vi "RPC_DAQV3.vi"(7 "address":string[](array[string])=["192.168.10.20", "192.168.10.35"], 8 "error in (no error)":errorcluster, 9 "stop":bool=TRUE, 10 "save data":bool=TRUE, 11 "SMA mode":bool) -> (0 "error out 3":errorcluster, 2 "csv path":path=path "G:/tdc/2017/data/test_20250827_105458.csv", 3 "rate":dbl)   [LabVIEW 2017]
uses:
  gloabal.vi
  <vilib>/Utility/file.llb/Write Delimited Spreadsheet (DBL).vi
  <vilib>/Utility/file.llb/Write Delimited Spreadsheet (I64).vi
panel:
  out "Module NO":i32
  out "数组":errorcluster[](array[cluster])
  out "大小 5":i32=2
  out "大小 4":i32=2
  in  "cpu":i32=7
  out "大小 3":i32=2
  out "大小 2":i32=2
  out "大小":i32=2
  out "name (unnamed) 6":string="03E8"
  out "fine time":u64=3
  out "PAD NO":u64
  out "hitmap":u64 format="%08b"
  out "Array":string[](array[string])
  out "rpc trigger rate":u32[](array[numeric])=[0, 1000, 1000, 1000, 0, 0, 0, 0, 0, 0, 0, 1000, 1000, 0, 0, 0, 0, 0, 0, 0]
  out "event":u32[](array[numeric])=[0, 760, 1760, 1000, 0, 0, 0, 0, 0, 0, 0, 160, 160, 0, 0, 0, 0, 0, 0, 0]
  in  "calib_file":path=path "G:/tdc/2017/data/112_20250410_codeDensity.csv" caption="文件路径 （空时为对话框）"
  in  "use_calib_file":bool
  in  "coarse counter width":u16(ring) items=["29", "48"]
  out "error out 5":errorcluster
  in  "timeout":dbl=30000.0
  out "Out":u8=3 format="%.0x"
  in  "factor":i32=128
  in  "displayCR":bool=TRUE
  in  "Counter Setting":dbl=100000.0 format="%#_13g"
  in  "replace dat":bool
  in  "append csv":bool=TRUE
  out "element":string
  out "time":u64=1011186851 format="%x"
  in  "UDP Config":bool
  in  "data  path":path=path "G:/tdc/2017/data"
  out "cal 2":u64[](graph)=[12185147, 13185148, 14185150, 15185152, 16185153, 17185155, 18185157, 19185159, 20185160, 21185162, 22185164, 23185165, 24185167, 25185169, 26185170, 27185172, 28185174, 29185176, 30185177, 31185179, 32185181, 33185183, 34185184, 35185186, 36185188, 37185189, 38185191, 39185192, 40185194, 41185196, 42185198, 43185199, 44185201, 45185203, 46185205, 47185206, 48185208, 49185210, 50185212, 51185213, 52185215, 53185216, 54185218, 55185220, 56185222, 57185223, 58185225, 59185227, 60185229, 61185230, 62185232, 63185234, 64185235, 65185237, 66185239, 67185240, 68185242, 69185244, 70185246, 71185247, 72185249, 73185251, 74185253, 75185254, 76185256, 77185257, 78185259, 79185261, 80185263, 81185264, 82185266, 83185268, 84185270, 85185271, 86185273, 87185275, 88185276, 89185278, 90185280, 91185281, 92185283, 93185285, 94185287, 95185288, 96185290, 97185292, 98185294, 99185295, 100185297, 101185299, 102185300, 103185302, 104185304, 105185305, 106185307, 107185309, 108185311, 109185312, 110185314, 111185316, 112185317, 113185319, 114185321, 115185323, 116185324, 117185326, 118185328, 119185329, 120185331, 121185333, 122185335, 123185336, 124185338, 125185340, 126185341, 127185343, 128185344, 129185347, 130185348, 131185350, 132185351, 133185353, 134185355, 135185357, 136185358, 137185360, 138185362, 139185364, 140185365, 141185367, 142185368, 143185370, 144185372, 145185374, 146185375, 147185377, 148185379, 149185381, 150185382, 151185384, 152185386, 153185388, 154185389, 155185391, 156185392, 157185394, 158185396, 159185398, 160185399, 161185401, 162185403, 163185404, 164185406, 165185408, 166185410, 167185412, 168185413, 169185415, 170185416, 171185418, 172185420, 173185422, 174185423, 175185425, 176185427, 177185428, 178185430, 179185432, 180185433, 181185435, 182185437, 183185439, 184185440, 185185442, 186185444, 187185446, 188185447, 189185449, 190185451, 191185452, 192185454, 193185456, 194185457, 195185459, 196185461, 197185463, 198185464, 199185466, 200185468, 201185469, 202185471, 203185473, 204185475, 205185476, 206185478, 207185480, 208185481, 209185483, 210185485, 211185486, 212185488, 213185490, 214185492, 215185493, 216185495, 217185496, 218185498, 219185500, 220185502, 221185503, 222185505, 223185507, 224185509, 225185510, 226185512, 227185514, 228185516, 229185517, 230185519, 231185520, 232185522, 233185524, 234185526, 235185527, 236185529, 237185531, 238185533, 239185534, 240185536, 241185537, 242185539, 243185541, 244185543, 245185544, 246185546, 247185548, 248185550, 249185551, 250185553, 251185555, 252185556, 253185558, 254185560, 255185561, 256185563, 257185565, 258185567, 259185568, 260185570, 261185572, 262185573, 263185575, 264185577, 265185579, 266185580, 267185582, 268185584, 269185585, 270185587, 271185589, 272185591, 273185592, 274185594, 275185596, 276185597, 277185599, 278185601, 279185602, 280185604, 281185606, 282185608, 283185609, 284185611, 285185613, 286185615, 287185616, 288185618, 289185620, 290185621, 291185623, 372185761, 373185763, 374185765, 375185766, 376185768, 377185770, 378185772, 379185773, 380185775, 381185776, 382185778, 383185780, 384185782, 385185783, 386185785, 387185787, 388185788, 389185790, 390185792, 391185793, 392185795, 393185797, 394185799, 395185800, 396185802, 397185804, 398185806, 399185807, 400185809, 401185811, 402185812, 403185814, 404185816, 405185817, 406185819, 407185821, 408185823, 409185824, 410185826, 411185828, 412185829, 413185831, 414185833, 415185835, 416185836, 417185838, 418185840, 419185841, 420185843, 421185845, 422185847, 423185848, 424185850, 425185852, 426185853, 427185855, 428185857, 429185859, 430185860, 431185862, 432185864, 433185865, 434185867, 435185869, 436185871, 437185872, 438185874, 439185876, 440185877, 441185879, 442185881, 443185882, 444185884, 445185886, 446185887, 447185889, 448185891, 449185893, 450185894, 451185896, 452185898, 453185900, 454185901, 455185903, 456185904, 457185906, 458185908, 459185910, 460185911, 461185913, 462185915, 463185917, 464185918, 465185920, 466185921, 467185923, 468185925, 469185927, 470185928, 471185930, 472185932, 473185934, 474185935, 475185937, 476185939, 477185940, 478185942, 479185944, 480185946, 481185947, 482185949, 483185951, 484185952, 485185954, 486185956, 487185958, 488185959, 489185961, 490185963, 491185964, 492185966, 493185968, 494185969, 495185971, 496185973, 497185975, 498185976, 499185978, 500185980, 501185981, 502185983, 503185985, 504185987, 505185988, 506185990, 507185992, 508185993, 509185995, 510185997, 511185999, 512186000, 513186002, 514186004, 515186005, 516186007, 517186009, 518186011, 519186012, 520186014, 521186016, 522186017, 523186019, 524186021, 525186022, 526186024, 527186026, 528186028, 529186029, 530186031, 531186033, 532186034, 533186036, 534186038, 535186040, 536186041, 537186043, 538186045, 539186046, 540186048, 541186050, 542186052, 543186053, 544186055, 545186056, 546186058, 547186060, 548186062, 549186063, 550186065, 551186067, 552186069, 553186070, 554186072, 555186074, 556186076, 557186077, 558186079, 559186080, 560186082, 561186084, 562186086, 563186087, 564186089, 565186091, 566186093, 567186094, 568186096, 569186097, 570186099, 571186101, 572186103, 573186104, 574186106, 575186108, 576186110, 577186111, 578186113, 579186115, 580186116, 581186118, 582186120, 583186121, 584186123, 585186125, 586186127, 587186128, 588186130, 589186132, 590186133, 591186135, 592186137, 593186139, 594186140, 595186142, 596186144, 597186145, 598186147, 599186149, 600186151, 601186152, 602186154, 603186156, 604186157, 605186159, 606186160, 607186163, 608186164, 609186166, 610186167, 611186169, 692186308, 693186309, 694186311, 695186313, 696186315, 697186316, 698186318, 699186319, 700186321, 701186323, 702186325, 703186326, 704186328, 705186330, 706186332, 707186333, 708186335, 709186336, 710186338, 711186340, 712186342, 713186343, 714186345, 715186347, 716186349, 717186350, 718186352, 719186354, 720186356, 721186357, 722186359, 723186360, 724186362, 725186364, 726186366, 727186367, 728186369, 729186371, 730186373, 731186374, 732186376, 733186378, 734186379, 735186381, 736186383, 737186384, 738186386, 739186388, 740186390, 741186391, 742186393, 743186395, 744186397, 745186398, 746186400, 747186401, 748186403, 749186405, 750186407, 751186408, 752186410, 753186412, 754186414, 755186415, 756186417, 757186419, 758186420, 759186422, 760186424, 761186425, 762186427, 763186429, 764186431, 765186432, 766186434, 767186436, 768186438, 769186439, 770186441, 771186443, 772186444, 773186446, 774186448, 775186449, 776186451, 777186453, 778186455, 779186456, 780186458, 781186460, 782186461, 783186463, 784186465, 785186467, 786186468, 787186470, 788186472, 789186473, 790186475, 791186477, 792186478, 793186480, 794186482, 795186484, 796186485, 797186487, 798186489, 799186491, 800186492, 801186494, 802186496, 803186497, 804186499, 805186501, 806186502, 807186504, 808186506, 809186508, 810186509, 811186511, 812186513, 813186514, 814186516, 815186518, 816186519, 817186521, 818186523, 819186525, 820186526, 821186528, 822186530, 823186532, 824186533, 825186535, 826186536, 827186538, 828186540, 829186542, 830186543, 831186545, 832186547, 833186548, 834186550, 835186552, 836186554, 837186556, 838186557, 839186559, 840186560, 841186562, 842186564, 843186566, 844186567, 845186569, 846186571, 847186572, 848186574, 849186576, 850186577, 851186579, 852186581, 853186583, 854186584, 855186586, 856186588, 857186590, 858186591, 859186593, 860186595, 861186596, 862186598, 863186600, 864186601, 865186603, 866186605, 867186607, 868186608, 869186610, 870186612, 871186613, 872186615, 873186617, 874186619, 875186620, 876186622, 877186624, 878186625, 879186627, 880186629, 881186631, 882186632, 883186634, 884186636, 885186637, 886186639, 887186641, 888186643, 889186644, 890186646, 891186648, 892186649, 893186651, 894186653, 895186655, 896186656, 897186658, 898186660, 899186661, 900186663, 901186664, 902186666, 903186668, 904186670, 905186672, 906186673, 907186675, 908186677, 909186678, 910186680, 911186682, 912186684, 913186685, 914186687, 915186688, 916186690, 917186692, 918186694, 919186695, 920186697, 921186699, 922186701, 923186702, 924186704, 925186706, 926186707, 927186709, 928186711, 929186712, 930186714, 931186716]
  in  "Thresholds (mV)":dbl[](array[numeric])=[580.0, 580.0, 580.0, 580.0, 600.0, 600.0, 600.0, 600.0, 580.0, 580.0, 600.0, 600.0, 600.0, 600.0, 600.0, 600.0, 580.0, 580.0, 600.0, 600.0, 600.0, 600.0, 600.0, 600.0, 580.0, 580.0, 600.0, 600.0, 600.0, 600.0, 600.0, 600.0, 600.0, 600.0, 600.0, 600.0, 600.0, 600.0, 600.0, 600.0, 600.0, 600.0, 600.0, 600.0, 600.0, 600.0, 600.0, 600.0, 600.0, 600.0, 600.0, 600.0, 600.0, 600.0, 600.0, 600.0, 600.0, 600.0, 600.0, 600.0, 600.0, 600.0, 600.0, 600.0]
  out "error out 2":errorcluster
  in  "display":bool=TRUE
  in  "Thresholds":dbl=-0.03
  in  "one key for threshold":bool=TRUE
  in  "RST":bool
  in  "通道数量":i32=10
  out "Cal Table":u32[](array[numeric])
  in  "channel for cal":i32
  out "Strip NO":u64
  out "Calibration Counter":i32=3364
  out "Event index":i32=97959
  out "cal":i64[](graph)
  out "error out":errorcluster
  out "appended path":path=path "G:/tdc/2017/data/test_20250827_105458.dat"
  in  "filename":string="test"
  in  "Events":i32=110000 min=1
  in  "timeout (ms)":i32=10000
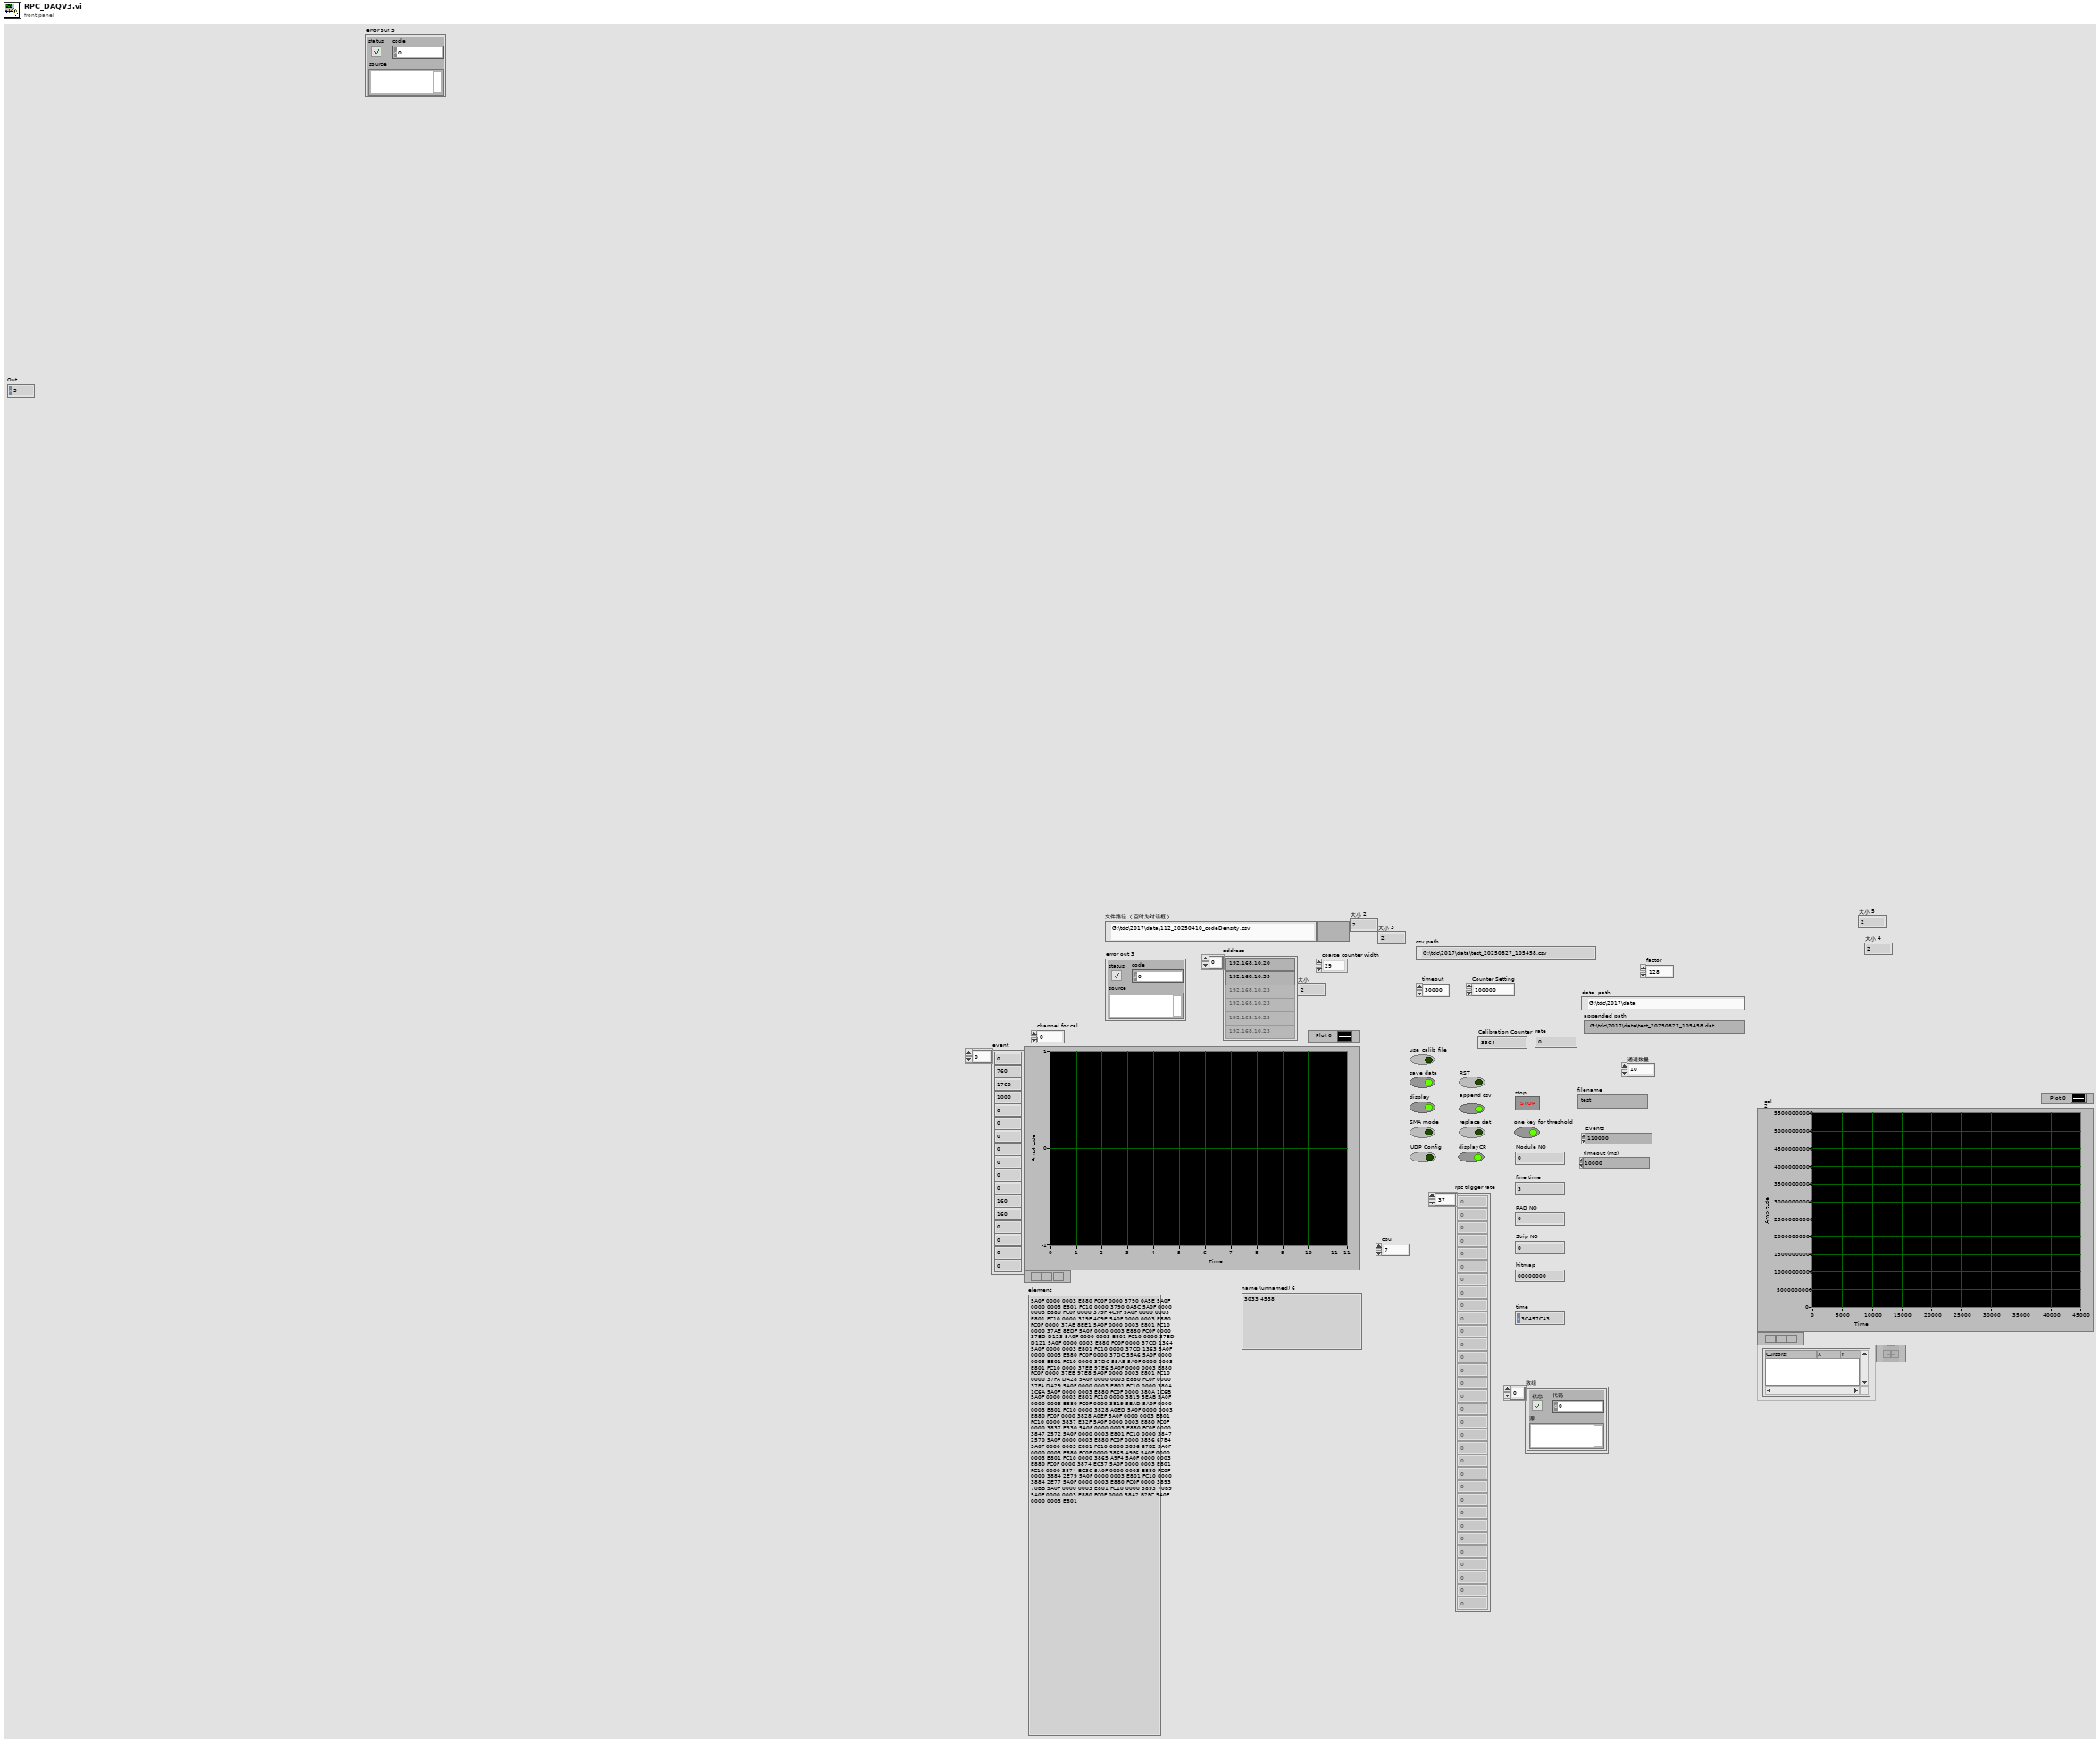
[diagram p1: front panel]
types:
  T1 = enum16{"open", "replace", "create", "open or create", "replace or create", "replace or create with confirmation"}
  T2 = enum16{"big-endian, network order", "native, host order", "little-endian"}
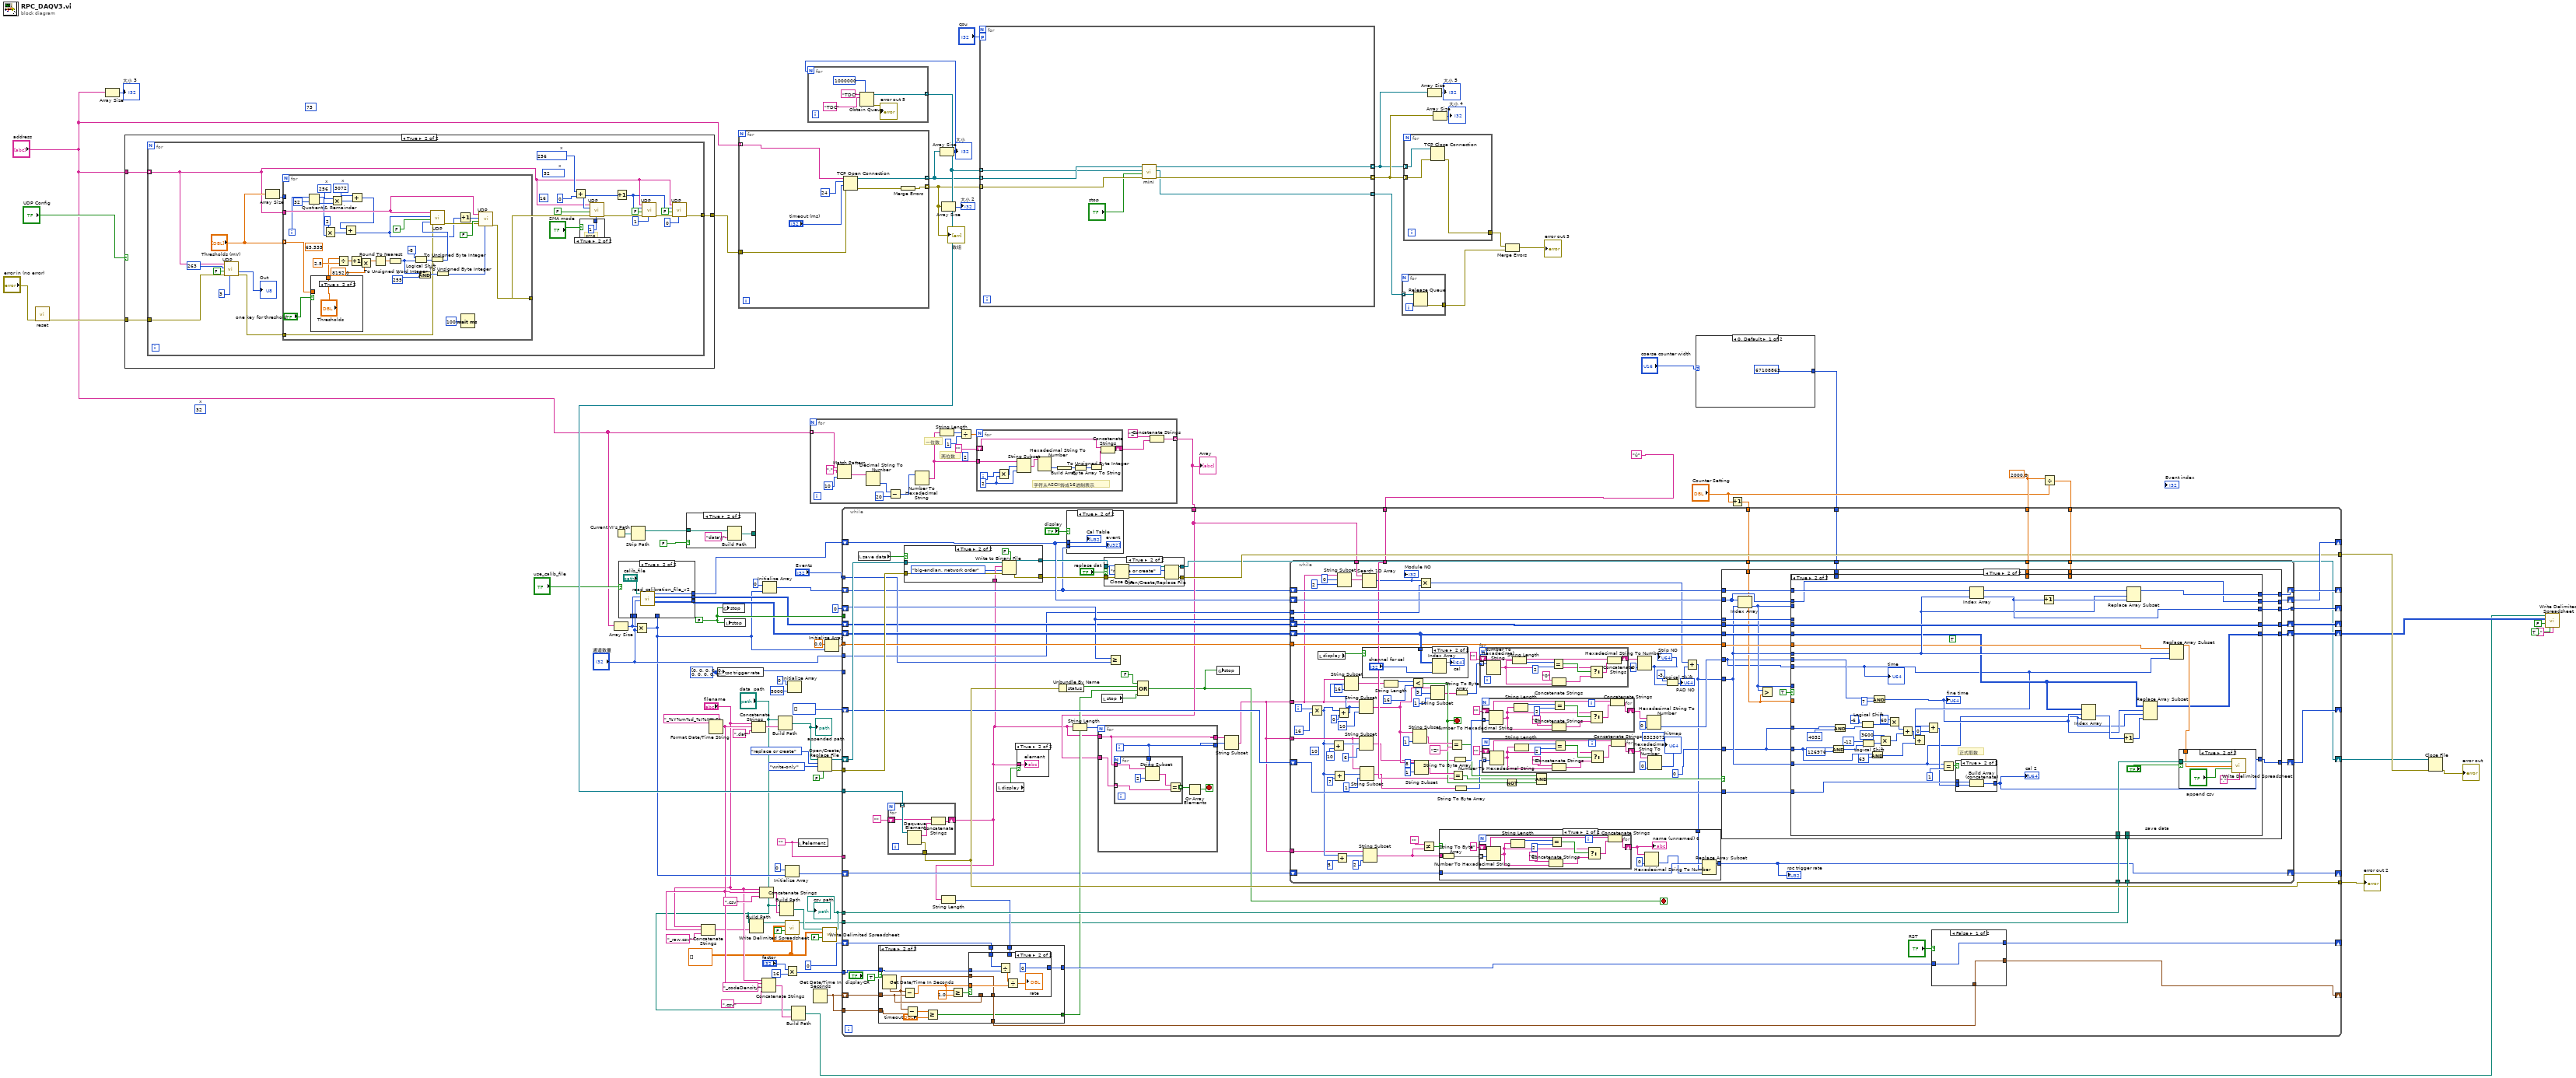
[diagram p0: block diagram]
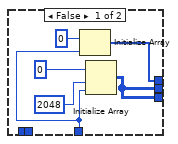
[diagram p2: hidden frame]
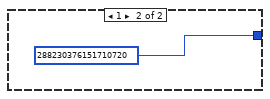
[diagram p3: hidden frame]
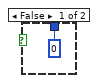
[diagram p5: hidden frame]
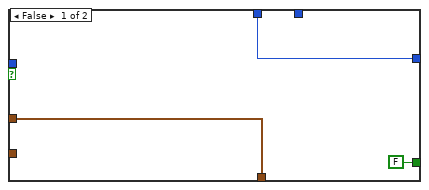
[diagram p11: hidden frame]
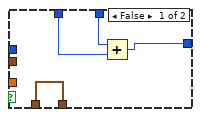
[diagram p12: hidden frame]
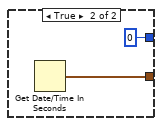
[diagram p14: hidden frame]
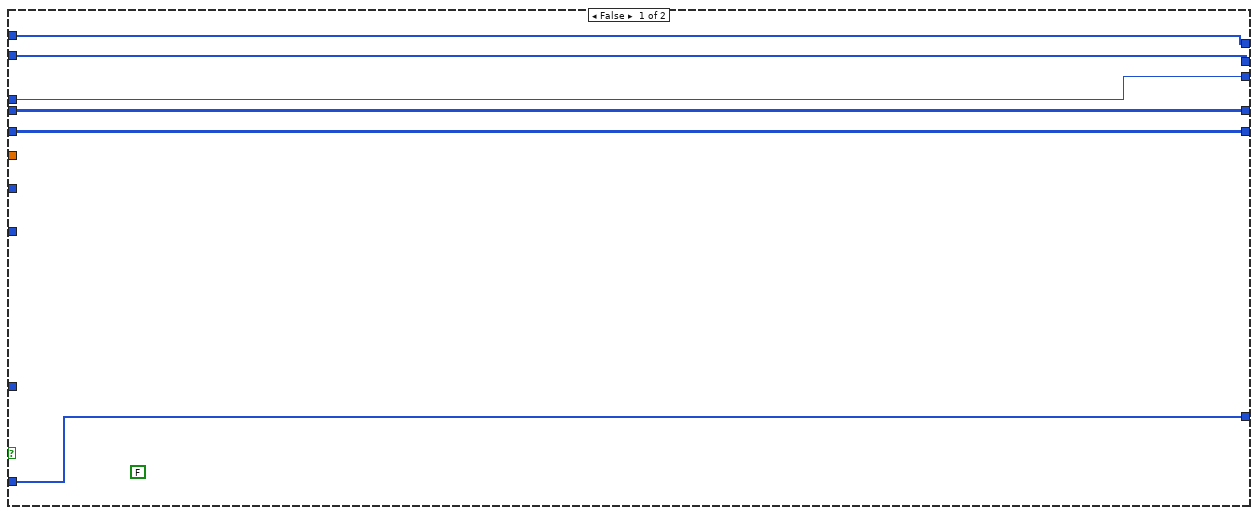
[diagram p17: hidden frame]
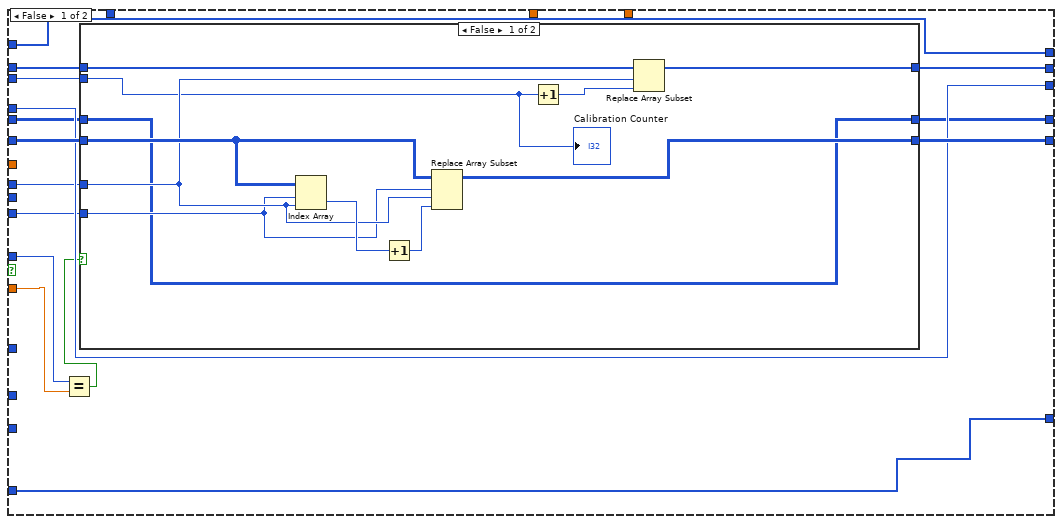
[diagram p18: hidden frame]
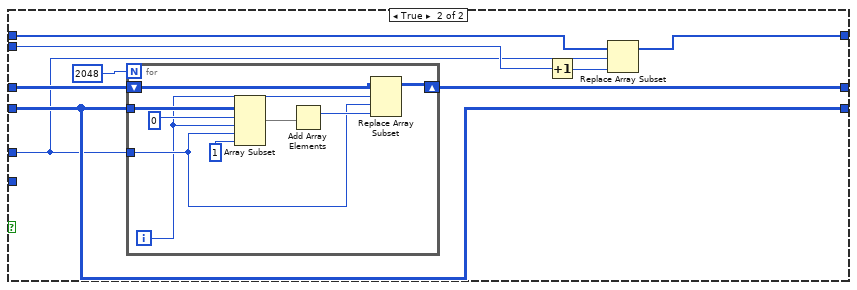
[diagram p19: hidden frame]
diagram:
  w24 = ""
  w25 = u32[] [0, 0, 0, 0, 0, 0, 0, 0, 0, 0, 0, 0, 0, 0, 0, 0, 0, 0, 0, 0, 0, 0, 0, 0, 0, 0, 0, 0, 0, 0, 0, 0, 0, 0, 0, 0, 0, 0, 0, 0, 0, 0, 0, 0, 0, 0, 0, 0, 0, 0, 0, 0, 0, 0, 0, 0, 0, 0, 0, 0, 0, 0, 0, 0] ("pmt trigger rate")
  (unwired) u32 73 ("Address")
  w56 = 2000.0 ("x")
  (unwired) u16 32  # x
  w38 = FALSE ("stop")
  w18 = dbl[][] [] ("2D data")
  n1 = call "reset.vi"("error in (no error)"="error in (no error)") -> ("error out"=w12:errorcluster)  [unwired: 10 in]
  n2 = Array Size(array="address") -> (size(s)=→"大小 3":i32)
  n3 = case shown="True" "UDP Config" {
    tunnel: "address" -> [_ w94]
    tunnel: [_ w95] -> w42
    tunnel: w12 -> [_ w93]
    frame False {
    }
    frame True {
      n4 = for {
        tunnel: [w101] -> w95
        tunnel: w94 -> [w99] mode=indexing
        tunnel: w93 -> [w96]
        (unwired) u16 32  # x
        (unwired) u32 16 ("Address")
        w112 = u16 256  # x
        n5 = call "UDP.vi"("In"=u8 3, "error in (no error)"=w96, "Read (TRUE)"=FALSE, "Address"=u32 263, "IP address"=w99) -> ("error out"=w107:errorcluster, "Out"=→"Out":u8)  [unwired: 3 in, 1 out]
        n6 = Array Size(array="Thresholds (mV)") -> (size(s)=w115:i32)
        n7 = for {
          tunnel: w99 -> [w151]
          tunnel: "Thresholds (mV)" -> [w138] mode=indexing
          tunnel: [w141] -> w118
          tunnel: w115 -> [_]
          tunnel: w107 -> [w125]
          i -> [w133]
          (unwired) 65.535 ("y")
          w134 = u16 3072  # x
          w135 = u16 256  # x
          w147 = u16 255  # x
          n8 = Quotient & Remainder(x=w133, y=32) -> (x-y*floor(x/y)=w127:i32, floor(x/y)=w136:i32)
          n9 = case shown="True" "one key for threshold" {
            tunnel: [w157 "Thresholds"] -> w139
            tunnel: w138 -> [w157 _]
            frame False {
            }
            frame True {
            }
          }
          n10 = Multiply(x=2, y=w127) -> (x*y=w128:i32)
          n11 = Multiply(x=w135, y=w136) -> (x*y=w130:i32)
          n12 = Divide(x=w139, y=2.5) -> (x/y=w154:dbl)
          n13 = Increment(x=w154) -> (x+1=w124:dbl)
          n14 = Add(x=w134, y=w130) -> (x+y=w129:i32)
          n15 = Add(x=w129, y=w128) -> (x+y=w132:i32)
          n16 = Multiply(x=w124, y=8192.0) -> (x*y=w123:dbl)
          n17 = Round To Nearest(number=w123) -> (nearest integer value=w152:dbl)
          n18 = To Unsigned Word Integer(number=w152) -> (unsigned 16bit integer=w143:u16)
          n19 = Logical Shift(y=i16 -8, x=w143) -> (x << y=w149:u16)
          n20 = And(x=w143, y=w147) -> (x .and. y?=w146:u16)
          n21 = To Unsigned Byte Integer(number=w149) -> (unsigned 8bit integer=w148:u8)
          n22 = call "UDP.vi"("In"=w148, "error in (no error)"=w125, "Read (TRUE)"=FALSE, "Address"=w132, "IP address"=w151) -> ("error out"=w142:errorcluster)  [unwired: 3 in, 2 out]
          n23 = To Unsigned Byte Integer(number=w146) -> (unsigned 8bit integer=w145:u8)
          n24 = Increment(x=w132) -> (x+1=w131:i32)
          n25 = Wait (ms)(milliseconds to wait=u32 100) -> ()  [unwired: 1 out]
          n26 = call "UDP.vi"("In"=w145, "error in (no error)"=w142, "Read (TRUE)"=FALSE, "Address"=w131, "IP address"=w151) -> ("error out"=w141:errorcluster)  [unwired: 3 in, 2 out]
        }
        n27 = Add(x=w112, y=u32 0 ("Address")) -> (x+y=w105:u32)
        n28 = case shown="True" "SMA mode" {
          tunnel: [u8 0 ("In") u8 1 ("In")] -> w117
          frame False {
          }
          frame True {
            # "sma"
          }
        }
        n29 = call "UDP.vi"("In"=w117, "error in (no error)"=w118, "Read (TRUE)"=FALSE, "Address"=w105, "IP address"=w99) -> ("error out"=w106:errorcluster)  [unwired: 3 in, 2 out]
        n30 = Increment(x=w105) -> (x+1=w98:u32)
        n31 = call "UDP.vi"("In"=u8 1, "error in (no error)"=w106, "Read (TRUE)"=FALSE, "Address"=w98, "IP address"=w99) -> ("error out"=w102:errorcluster)  [unwired: 3 in, 2 out]
        n32 = call "UDP.vi"("In"=u8 0, "error in (no error)"=w102, "Read (TRUE)"=FALSE, "Address"=w98, "IP address"=w99) -> ("error out"=w101:errorcluster)  [unwired: 3 in, 2 out]
      }
    }
  }
  n33 = Current VI's Path() -> (path=w87:path)
  n34 = Array Size(array="address") -> (size(s)=w30:i32)
  n35 = Strip Path(path=w87) -> (stripped path=w86:path)  [unwired: 1 out]
  n36 = Multiply(x=w30, y="通道数量") -> (x*y=w27:i32)
  n37 = case shown="True" "use_calib_file" {
    tunnel: w27 -> [w162 _]
    tunnel: [w159 w170] -> w33
    tunnel: [w159 w169] -> w32
    tunnel: [w160 w168] -> w31
    tunnel: w30 -> [_ w167]
    tunnel: "通道数量" -> [_ w166]
    frame False {
      n38 = Initialize Array(u32 0 ("element"), w162) -> (w160:u32[])
      n39 = Initialize Array(u32 0 ("element"), 2048 ("dimension size"), w162) -> (w159:u32[][])
    }
    frame True {
      n40 = call "read_calibration_file_v2.vi"("通道数量"=w166, "板子数量"=w167, "file path (dialog if empty)"="calib_file") -> ("code_density"=w170:i64[][], "accumulation"=w169:u32[][], "Cal Table"=w168:u32[])  [unwired: 5 in, 1 out]
    }
  }
  n41 = case shown="True" FALSE {
    tunnel: w86 -> [w171 w173]
    tunnel: [w171 w172] -> _
    frame False {
    }
    frame True {
      n42 = Build Path(base path=w173, name or relative path="data\\") -> (appended path=w172:path)
    }
  }
  n43 = Format Date/Time String(time format string (%c)="_%Y%m%d_%I%M%S") -> (date/time string=w22:string)  [unwired: 2 in]
  n44 = Concatenate Strings("filename", w22, "_raw.csv") -> (w20:string)
  n45 = local write "rpc trigger rate"(w25) -> ()
  n46 = global write "gloabal.vi" "stop"(w38) -> ()
  n47 = local write "stop"(w38) -> ()
  n48 = for {
    tunnel: "address" -> [w180] mode=indexing
    tunnel: [w179] -> w10 mode=indexing
    tunnel: [w177] -> w11 mode=indexing
    tunnel: w42 -> [w176]
    n49 = TCP Open Connection(address=w180, remote port or service name=u16 24 ("port"), timeout ms (60000)="timeout (ms)", error in (no error)=w176) -> (connection ID=w179:refnum<k5>, error out=w178:errorcluster)  [unwired: 1 in]
    n50 = Merge Errors(w178) -> (w177:errorcluster)
  }
  "数组" <- w11
  n51 = Build Path(base path="data  path", name or relative path=w20) -> (appended path=w15:path)
  n52 = Concatenate Strings("filename", w22, ".dat") -> (w85:string)
  n53 = Concatenate Strings("filename", w22, ".csv") -> (w75:string)
  n54 = Concatenate Strings("filename", w22, "_codeDensity" ("string"), ".csv") -> (w68:string)
  n55 = Initialize Array(u32 0 ("element"), w27) -> (w74:u32[])
  n56 = Build Path(base path="data  path", name or relative path=w85) -> (appended path=w84:path)
  "appended path" <- w84
  n57 = Build Path(base path="data  path", name or relative path=w75) -> (appended path=w73:path)
  n58 = Initialize Array(u32 0 ("element"), w27) -> (w26:u32[])
  n59 = call-poly <vilib>:"Write Delimited Spreadsheet.vi"("file path (dialog if empty)"=w15, "2D data"=w18, "append to file? (new file:F)"=FALSE) -> ("new file path (Not A Path if cancelled)"=w16:path)  [unwired: 11 in, 1 out]
  n60 = Multiply(x="factor", y=16) -> (x*y=w49:i32)
  n61 = Initialize Array(u32 0 ("element"), 5000 ("dimension size")) -> ()  [unwired: 1 out]
  n62 = Build Path(base path="data  path", name or relative path=w68) -> (appended path=w65:path)
  n63 = local write "element"(w24) -> ()
  n64 = for {
    tunnel: [w183] -> w46 mode=indexing
    tunnel: "address" -> [w182] mode=indexing
    (unwired) 2 ("y")
    # "一位数"
    # "两位数"
    n65 = Match Pattern(string=w182, regular expression="." ("search string"), offset (0)=10) -> (after substring=w189:string)  [unwired: 3 out]
    n66 = Decimal String To Number(string=w189) -> (number=w186:i32)  [unwired: 2 in, 1 out]
    n67 = Subtract(x=w186, y=20) -> (x-y=w185:i32)
    n68 = Number To Hexadecimal String(2:w185) -> (0:w188:string)  [unwired: 1 in]
    n69 = String Length(string=w188) -> (length=w194:i32)
    n70 = Divide(x=w194, y=1) -> (x/y=w195:dbl)
    n71 = for {
      N: w195 -> [_]
      shift-right: [w207] -> w184
      shift-left: "" ("format string") -> [w206]
      tunnel: w188 -> [w197]
      i -> [w205]
      w199 = 2 ("y")
      # "字符从ASCII转成16进制表示"
      n72 = Multiply(x=w205, y=w199) -> (x*y=w198:i32)
      n73 = String Subset(string=w197, offset (0)=w198, length (rest)=w199) -> (substring=w200:string)
      n74 = Hexadecimal String To Number(string=w200) -> (number=w204:u32)  [unwired: 2 in, 1 out]
      n75 = Build Array(w204) -> (w203:u32[])
      n76 = To Unsigned Byte Integer(number=w203) -> (unsigned 8bit integer=w202:u8[])
      n77 = Byte Array To String(unsigned byte array=w202) -> (string=w201:string)
      n78 = Concatenate Strings(w206, w201) -> (w207:string)
    }
    n79 = Concatenate Strings("Z", w184) -> (w183:string)
  }
  "Array" <- w46
  n80 = Get Date/Time In Seconds() -> (seconds since 1Jan1904=w45:timestamp)
  n81 = Open/Create/Replace File(file path (use dialog)=w84, operation (0:open)=T1."replace or create", access (0:read/write)=enum16{"read/write", "read-only", "write-only"}."write-only", disable buffering (F)=FALSE) -> (refnum out=w89:refnum<file>, error out=w88:errorcluster)  [unwired: 2 in, 1 out]
  n82 = call-poly <vilib>:"Write Delimited Spreadsheet.vi"("file path (dialog if empty)"=w73, "2D data"=w18, "append to file? (new file:F)"=FALSE) -> ("new file path (Not A Path if cancelled)"=w37:path)  [unwired: 11 in, 1 out]
  "csv path" <- w37
  n83 = Initialize Array(0.0, w27) -> (w61:dbl[])
  n84 = Array Size(array=w10) -> (size(s)=w2:i32)
  "大小" <- w2
  n85 = for {
    N: w2 -> [_]
    tunnel: [w208] -> w43 mode=indexing
    n86 = Obtain Queue(max queue size (-1, unlimited)=1000000, name (unnamed)="TDC", element data type="TDC" ("name (unnamed)")) -> (queue out=w208:refnum<queue>, error out=→"error out 5":errorcluster)  [unwired: 2 in, 1 out]
  }
  n87 = Array Size(array=w11) -> (size(s)=→"大小 2":i32)
  n88 = for {
    tunnel: w10 -> [w219] mode=indexing
    tunnel: w11 -> [w218] mode=indexing
    tunnel: [w217] -> w3 mode=indexing
    tunnel: [w216] -> w5 mode=indexing
    tunnel: w43 -> [w215] mode=indexing
    tunnel: [w214] -> w44 mode=indexing
    workers-P: "cpu" -> [_]
    n89 = call "mini.vi"("error in (no error)"=w218, "stop"="stop", "queue out 2"=w215, "connection ID 2"=w219) -> ("error out 3"=w216:errorcluster, "queue out"=w214:refnum<queue>, "connection ID"=w217:refnum<k5>)  [unwired: 5 in]
  }
  n90 = for {
    tunnel: w44 -> [w221] mode=indexing
    tunnel: [w220] -> w40
    n91 = Release Queue(queue=w221) -> (error out=w220:errorcluster)  [unwired: 2 in, 2 out]
  }
  n92 = for {
    tunnel: w3 -> [w224] mode=indexing
    tunnel: w5 -> [w223] mode=indexing
    tunnel: [w222] -> w41
    n93 = TCP Close Connection(connection ID=w224, error in (no error)=w223) -> (error out=w222:errorcluster)  [unwired: 1 in, 1 out]
  }
  n94 = Array Size(array=w3) -> (size(s)=→"大小 5":i32)
  n95 = Array Size(array=w5) -> (size(s)=→"大小 4":i32)
  n96 = Merge Errors(w41, w40) -> (→"error out 3":errorcluster)
  n97 = case shown="0, Default" "coarse counter width" {
    tunnel: [u64 67108863 ("port") u64 288230376151710720 ("port")] -> w35
    frame 0, Default {
    }
    frame 1 {
    }
  }
  n98 = Increment(x="Counter Setting") -> (x+1=w52:dbl)
  n99 = Divide(x=w56, y="Counter Setting") -> (x/y=w55:dbl)
  n100 = while {
    tunnel: w88 -> [w285]
    tunnel: [w266] -> w62
    tunnel: [w255] -> w81
    shift-right: [w282] -> w66
    shift-left: w33 -> [w283]
    tunnel: "Events" -> [w280]
    shift-right: [w279] -> _
    shift-left: w74 -> [w233]
    shift-right: [w278] -> _
    shift-left: u32 0 ("element") -> [w277]
    shift-right: [w276] -> _
    shift-left: w31 -> [w268]
    shift-right: [w270] -> _
    shift-left: w32 -> [w275]
    tunnel: w37 -> [w262]
    shift-right: [w274] -> _
    shift-left: 0 -> [w249]
    shift-right: [w272] -> _
    shift-left: w45 -> [w271]
    tunnel: w38 -> [_]
    tunnel: w43 -> [w267]
    shift-right: [w263] -> _
    shift-left: u64[] [] -> [w264]
    tunnel: w46 -> [w237]
    tunnel: w56 -> [w260]
    tunnel: w55 -> [w259]
    shift-right: [w254] -> w54
    shift-left: w89 -> [w284]
    tunnel: w52 -> [w253]
    tunnel: w49 -> [w246]
    tunnel: "ü" ("format string") -> [w244]
    tunnel: w45 -> [w243]
    tunnel: "通道数量" -> [w238]
    tunnel: w35 -> [w234]
    shift-right: [w230] -> _
    shift-left: w26 -> [w231]
    tunnel: w25 -> [_]
    tunnel: w24 -> [_]
    tunnel: w16 -> [w229]
    tunnel: w61 -> [w281]
    stop <- w236 stop-if-true
    n101 = local read "save data"() -> (w248:bool)
    n102 = for {
      tunnel: w267 -> [w290] mode=indexing
      tunnel: [w289] -> w266
      shift-right: [w288] -> w227
      shift-left: "" -> [w286]
      n103 = Dequeue Element(queue=w290) -> (element=w287:string, error out=w289:errorcluster)  [unwired: 2 in, 2 out]
      n104 = Concatenate Strings(w286, w287) -> (w288:string)
    }
    n105 = case shown="True" w248 {
      tunnel: w285 -> [w303 w311]
      tunnel: w284 -> [w304 w310]
      tunnel: w227 -> [_ w308]
      tunnel: [w304 w307] -> w258
      tunnel: [w303 w306] -> w256
      frame False {
      }
      frame True {
        n106 = Write to Binary File(file (use dialog)=w310, data=w308, error in=w311, 5:FALSE ("prepend array or string size? (T)"), 9:T2."big-endian, network order" ("byte order (0:big-endian, network order)")) -> (refnum out=w307:refnum<file>, error out=w306:errorcluster)  [unwired: 1 in, 1 out]
      }
    }
    n107 = String Length(string=w227) -> (length=w250:i32)
    n108 = case shown="True" TRUE {
      tunnel: w271 -> [w323 w333]
      tunnel: [w323 w334] -> w252
      tunnel: w249 -> [w322 w332]
      tunnel: w250 -> [_ w331]
      tunnel: [w322 w330] -> w251
      tunnel: w246 -> [_ w329]
      tunnel: w243 -> [_ w327]
      tunnel: [FALSE w324] -> w242
      frame False {
      }
      frame True {
        n109 = Get Date/Time In Seconds() -> (seconds since 1Jan1904=w328:timestamp)
        n110 = Subtract(x=w328, y=w333) -> (x-y=w336:dbl)
        n111 = Subtract(x=w328, y=w327) -> (x-y=w326:dbl)
        n112 = Greater Or Equal?(x=w326, y="timeout") -> (x >= y?=w324:bool)
        n113 = Greater Or Equal?(x=w336, y=1.0) -> (x >= y?=w337:bool)
        n114 = case shown="True" w337 {
          tunnel: w336 -> [_ w348]
          tunnel: w328 -> [_ w346]
          tunnel: [w341 w346] -> w334
          tunnel: w333 -> [w341 _]
          tunnel: w332 -> [w340 w343]
          tunnel: w331 -> [w339 _]
          tunnel: [w338 0] -> w330
          tunnel: w329 -> [_ w342]
          frame False {
            n115 = Add(x=w339, y=w340) -> (x+y=w338:i32)
          }
          frame True {
            n116 = Divide(x=w343, y=w342) -> (x/y=w345:dbl)
            n117 = Divide(x=w345, y=w348) -> (x/y=→"rate":dbl)
          }
        }
      }
    }
    n118 = local read "display"() -> (w247:bool)
    n119 = case shown="True" w247 {
      tunnel: w227 -> [_ w302]
      frame False {
      }
      frame True {
        "element" <- w302
      }
    }
    n120 = Unbundle By Name(w266) -> ("status"=w265:bool)
    n121 = case shown="True" "display" {
      tunnel: w268 -> [_ w350]
      tunnel: w233 -> [_ w349]
      frame False {
      }
      frame True {
        "Cal Table" <- w350
        "event" <- w349
      }
    }
    n122 = String Length(string=w227) -> (length=w241:i32)
    n123 = for {
      N: w241 -> [_]
      tunnel: w227 -> [w295]
      tunnel: [w295] -> w240
      tunnel: [w294] -> w239
      tunnel: w237 -> [w293]
      i -> [w294]
      stop <- w292 stop-if-true
      n124 = for {
        tunnel: [w300] -> w291 mode=indexing
        tunnel: w295 -> [w299]
        tunnel: w294 -> [w298]
        tunnel: w293 -> [w296] mode=indexing
        n125 = String Subset(string=w299, offset (0)=w298, length (rest)=2 ("length (rest)")) -> (substring=w297:string)
        n126 = Equal?(x=w297, y=w296) -> (x = y?=w300:bool)
      }
      n127 = Or Array Elements(Boolean array=w291) -> (logical OR=w292:bool)
    }
    n128 = local read "stop"() -> (w235:bool)
    n129 = case shown="True" "replace dat" {
      tunnel: w258 -> [w313 w319]
      tunnel: [w313 w318] -> w254
      tunnel: w256 -> [w312 w315]
      tunnel: [w312 w314] -> w255
      frame False {
      }
      frame True {
        n130 = Close File(refnum=w319, error in=w315) -> (path=w320:path, error out=w316:errorcluster)
        n131 = Open/Create/Replace File(file path (use dialog)=w320, error in=w316, operation (0:open)=T1."replace or create") -> (refnum out=w318:refnum<file>, error out=w314:errorcluster)  [unwired: 3 in, 1 out]
      }
    }
    n132 = Greater Or Equal?(x=w277, y=w280) -> ()  [unwired: 1 out]
    n133 = Compound Arithmetic op=OR(FALSE ("x"), w265, w242, w235) -> (w236:bool)
    n134 = global write "gloabal.vi" "stop"(w236) -> ()
    n135 = String Subset(string=w240, offset (0)=w239) -> (substring=w232:string)  [unwired: 1 in]
    n136 = while {
      tunnel: w232 -> [w366]
      shift-right: [w442] -> w282
      shift-left: w283 -> [w441]
      shift-right: [w437] -> w279
      shift-left: w233 -> [w436]
      tunnel: [w435] -> w278
      tunnel: w277 -> [w434]
      shift-right: [w432] -> w276
      shift-left: w268 -> [w433]
      tunnel: w262 -> [w430]
      shift-right: [w429] -> w270
      shift-left: w275 -> [w401]
      shift-right: [w426] -> w263
      shift-left: w264 -> [w427]
      tunnel: w232 -> [w395]
      tunnel: w260 -> [w407]
      tunnel: w259 -> [w406]
      tunnel: w253 -> [w400]
      tunnel: w244 -> [w390]
      tunnel: w238 -> [w381]
      tunnel: w237 -> [w380]
      tunnel: w234 -> [w378]
      tunnel: w232 -> [w371]
      shift-right: [w363] -> w230
      shift-left: w231 -> [w373]
      tunnel: w229 -> [w368]
      tunnel: w281 -> [w440]
      i -> [w443]
      stop <- w403 stop-if-true
      (unwired) 10 ("length (rest)")
      (unwired) u64 8323072 ("port")
      n137 = Multiply(x=w443, y=16 ("length (rest)")) -> (x*y=w374:i32)
      n138 = local read "display"() -> (w428:bool)
      n139 = Add(x=w374, y=10 ("length (rest)")) -> (x+y=w418:i32)
      n140 = Add(x=w374, y=7 ("length (rest)")) -> (x+y=w397:i32)
      n141 = Add(x=w374, y=5 ("length (rest)")) -> (x+y=w376:i32)
      n142 = Add(x=w374, y=0 ("length (rest)")) -> (x+y=w405:i32)
      n143 = String Subset(string=w366, offset (0)=0, length (rest)=2 ("length (rest)")) -> (substring=w355:string)
      n144 = String Subset(string=w366, offset (0)=w405, length (rest)=16 ("y")) -> (substring=w358:string)
      n145 = String Subset(string=w366, offset (0)=w405, length (rest)=10 ("length (rest)")) -> (substring=w365:string)
      n146 = String Subset(string=w395, offset (0)=w418, length (rest)=6 ("length (rest)")) -> (substring=w364:string)
      n147 = String Subset(string=w395, offset (0)=w397, length (rest)=1 ("length (rest)")) -> (substring=w386:string)
      n148 = Search 1D Array(1D array=w380, element=w355) -> (index of element=w382:i32)  [unwired: 1 in]
      "Module NO" <- w382
      n149 = case shown="True" w428 {
        tunnel: w441 -> [_ w488]
        frame False {
        }
        frame True {
          n150 = Index Array(array=w488, index (col)="channel for cal") -> (element=→"cal":i64[])  [unwired: 1 in]
        }
      }
      n151 = String Subset(string=w371, offset (0)=w376, length (rest)=2 ("length (rest)")) -> (substring=w356:string)
      n152 = String Length(string=w358) -> (length=w439:i32)
      n153 = Less?(x=w439, y=16) -> (x < y?=w403:bool)
      n154 = String Subset(string=w365, length (rest)=1 ("length (rest)")) -> (substring=w423:string)  [unwired: 1 in]
      n155 = String Subset(string=w365, offset (0)=8, length (rest)=1 ("length (rest)")) -> (substring=w408:string)
      n156 = Multiply(x=w382, y=w381) -> (x*y=w379:i32)
      n157 = Not Equal?(x="", y=w356) -> (x != y?=w370:bool)
      n158 = String Subset(string=w365, offset (0)=9, length (rest)=1 ("length (rest)")) -> (substring=w387:string)
      n159 = Equal?(x=w423, y="Z" ("format string")) -> (x = y?=w409:bool)
      n160 = Equal?(x=w408, y=w390) -> (x = y?=w362:bool)
      n161 = String To Byte Array(string=w364) -> (unsigned byte array=w415:u8[])
      n162 = String To Byte Array(string=w386) -> (unsigned byte array=w391:u8[])
      n163 = String To Byte Array(string=w387) -> (unsigned byte array=w444:u8[])
      n164 = for {
        shift-right: [w622] -> w412
        shift-left: "" ("format string") -> [w619]
        tunnel: w444 -> [w623] mode=indexing
        n165 = Number To Hexadecimal String(2:w623) -> (0:w615:string)  [unwired: 1 in]
        n166 = String Length(string=w615) -> (length=w621:i32)
        n167 = Equal?(x=w621, y=2) -> (x = y?=w618:bool)
        n168 = Concatenate Strings("0" ("format string"), w615) -> (w617:string)
        n169 = Select(t=w615, s=w618, f=w617) -> (s? t:f=w614:string)
        n170 = Concatenate Strings(w619, w614) -> (w622:string)
      }
      n171 = for {
        shift-right: [w484] -> w413
        shift-left: "" ("format string") -> [w476]
        tunnel: w415 -> [w485] mode=indexing
        n172 = Number To Hexadecimal String(2:w485) -> (0:w478:string)  [unwired: 1 in]
        n173 = String Length(string=w478) -> (length=w483:i32)
        n174 = Concatenate Strings("0" ("format string"), w478) -> (w480:string)
        n175 = Equal?(x=w483, y=2) -> (x = y?=w481:bool)
        n176 = Select(t=w478, s=w481, f=w480) -> (s? t:f=w477:string)
        n177 = Concatenate Strings(w476, w477) -> (w484:string)
      }
      n178 = for {
        shift-right: [w474] -> w394
        shift-left: "" ("format string") -> [w466]
        tunnel: w391 -> [w475] mode=indexing
        n179 = Number To Hexadecimal String(2:w475) -> (0:w468:string)  [unwired: 1 in]
        n180 = String Length(string=w468) -> (length=w473:i32)
        n181 = Concatenate Strings("0" ("format string"), w468) -> (w470:string)
        n182 = Equal?(x=w473, y=2) -> (x = y?=w471:bool)
        n183 = Select(t=w468, s=w471, f=w470) -> (s? t:f=w467:string)
        n184 = Concatenate Strings(w466, w467) -> (w474:string)
      }
      n185 = Not(x=w403) -> (.not. x?=w402:bool)
      n186 = Compound Arithmetic op=AND(w409, w362, w402) -> (w421:bool)
      n187 = Hexadecimal String To Number(string=w412, default (0uL)=u64 0 ("default (0 U32)")) -> (number=w359:u64)  [unwired: 1 in, 1 out]
      "Strip NO" <- w359
      n188 = Hexadecimal String To Number(string=w413, default (0uL)=u64 0 ("default (0 U32)")) -> (number=w385:u64)  [unwired: 1 in, 1 out]
      n189 = Hexadecimal String To Number(string=w394, default (0uL)=u64 0 ("default (0 U32)")) -> (number=→"hitmap":u64)  [unwired: 1 in, 1 out]
      n190 = Logical Shift(y=i16 -3, x=w359) -> (x << y=w357:u64)
      "PAD NO" <- w357
      n191 = Add(x=w379, y=w357) -> (x+y=w372:u64)
      n192 = case shown="True" w370 {
        tunnel: w373 -> [w446 w452]
        tunnel: w372 -> [_ w450]
        tunnel: [w446 w449] -> w363
        tunnel: w356 -> [_ w448]
        frame False {
        }
        frame True {
          n193 = String To Byte Array(string=w448) -> (unsigned byte array=w453:u8[])
          n194 = for {
            shift-right: [w464] -> w447
            shift-left: "" ("format string") -> [w456]
            tunnel: w453 -> [w465] mode=indexing
            n195 = Number To Hexadecimal String(2:w465) -> (0:w458:string)  [unwired: 1 in]
            n196 = String Length(string=w458) -> (length=w463:i32)
            n197 = Concatenate Strings("0" ("format string"), w458) -> (w460:string)
            n198 = Equal?(x=w463, y=2) -> (x = y?=w461:bool)
            n199 = Select(t=w458, s=w461, f=w460) -> (s? t:f=w457:string)
            n200 = Concatenate Strings(w456, w457) -> (w464:string)
          }
          "name (unnamed) 6" <- w447
          n201 = Hexadecimal String To Number(string=w447, default (0uL)=u64 0 ("default (0 U32)")) -> (number=w451:u64)  [unwired: 1 in, 1 out]
          n202 = Replace Array Subset(array=w452, new element=w451, index=w450) -> (w449:u32[])
        }
      }
      "rpc trigger rate" <- w363
      n203 = case shown="True" w421 {
        tunnel: w385 -> [_ w495]
        tunnel: w434 -> [w492 w512]
        tunnel: w441 -> [w494 w518]
        tunnel: [w494 w517] -> w442
        tunnel: w440 -> [_ w516]
        tunnel: w372 -> [_ w503]
        tunnel: w436 -> [w493 w515]
        tunnel: [w493 w514] -> w437
        tunnel: [w492 w513] -> w435
        tunnel: w433 -> [w491 w511]
        tunnel: [w491 w510] -> w432
        tunnel: w401 -> [w490 w508]
        tunnel: [w490 w507] -> w429
        tunnel: w430 -> [_ w506]
        tunnel: w427 -> [w489 w505]
        tunnel: [w489 w504] -> w426
        tunnel: w407 -> [_ w502]
        tunnel: w406 -> [_ w501]
        tunnel: w400 -> [_ w500]
        tunnel: u64 0 ("default (0 U32)") -> [_ w499]
        tunnel: w378 -> [_ w498]
        tunnel: w368 -> [_ w497]
        frame False {
          (unwired) FALSE
        }
        frame True {
          n204 = Index Array(array=w511, index=w503) -> (element=w509:u32)
          n205 = Greater?(x=w509, y=w500) -> ()  [unwired: 1 out]
          n206 = case shown="True" TRUE {
            tunnel: w518 -> [w533 w567]
            tunnel: [w532 w565] -> w517
            tunnel: w495 -> [w525 w566]
            tunnel: w516 -> [_ w573]
            tunnel: w512 -> [w530 _]
            tunnel: w503 -> [w528 w574]
            tunnel: w515 -> [w531 w605]
            tunnel: [w531 w604] -> w514
            tunnel: [w530 w602] -> w513
            tunnel: w509 -> [w526 _]
            tunnel: w511 -> [w529 w601]
            tunnel: [w527 w601] -> w510
            tunnel: w509 -> [w523 _]
            tunnel: w500 -> [w520 _]
            tunnel: w508 -> [w522 w600]
            tunnel: [w521 w600] -> w507
            tunnel: w506 -> [_ w599]
            tunnel: w505 -> [w519 w596]
            tunnel: [w519 w595] -> w504
            tunnel: w503 -> [_ w563]
            tunnel: w502 -> [_ _]
            tunnel: w501 -> [_ _]
            tunnel: w499 -> [_ w589]
            tunnel: w499 -> [_ w578]
            tunnel: w495 -> [_ w572]
            tunnel: w498 -> [_ _]
            tunnel: w497 -> [_ _]
            frame False {
              n207 = Equal?(x=w523, y=w520) -> (x = y?=w524:bool)
              n208 = case shown="False" w524 {
                tunnel: w533 -> [w544 w550]
                tunnel: [w542 w550] -> w532
                tunnel: w529 -> [w540 w548]
                tunnel: w528 -> [w539 w545]
                tunnel: [w537 w547] -> w527
                tunnel: w526 -> [w536 w546]
                tunnel: w525 -> [w535 _]
                tunnel: w522 -> [w534 w552]
                tunnel: [w534 w551] -> w521
                frame False {
                  n209 = Index Array(array=w544, index (row)=w535, index (col)=w539) -> (element=w543:i64)
                  n210 = Increment(x=w543) -> (x+1=w541:i64)
                  n211 = Replace Array Subset(array=w544, new element=w541, index (row)=w535, index (col)=w539) -> (w542:i64[][])
                  n212 = Increment(x=w536) -> (x+1=w538:u32)
                  n213 = Replace Array Subset(array=w540, new element=w538, index=w539) -> (w537:u32[])
                  "Calibration Counter" <- w536
                }
                frame True {
                  n214 = for {
                    N: 2048 -> [_]
                    tunnel: w550 -> [w562]
                    tunnel: w545 -> [w555]
                    shift-right: [w557] -> w551
                    shift-left: w552 -> [w558]
                    i -> [w554]
                    n215 = Array Subset(array=w562, index (row)=0 ("索引"), length (row)=w554, index (col)=w555, length (col)=1 ("长度")) -> (w559:i64[][])
                    n216 = Add Array Elements(numeric array=w559) -> (sum=w556:i64)
                    n217 = Replace Array Subset(array=w558, new element=w556, index (row)=w554, index (col)=w555) -> (w557:u32[][])
                  }
                  n218 = Increment(x=w546) -> (x+1=w549:u32)
                  n219 = Replace Array Subset(array=w548, new element=w549, index=w545) -> (w547:u32[])
                }
              }
            }
            frame True {
              (unwired) TRUE
              # "正式取数"
              n220 = And(x=w578, y=u64 126976 ("port")) -> (x .and. y?=w586:u64)
              n221 = And(x=w589, y=u64 4032 ("port")) -> (x .and. y?=w592:u64)
              n222 = Logical Shift(y=i16 -6, x=w592) -> (x << y=w577:u64)
              n223 = Logical Shift(y=i16 -12, x=w586) -> (x << y=w585:u64)
              n224 = And(x=w578, y=u64 63 ("port")) -> (x .and. y?=w575:u64)
              n225 = And(x=w572, y=u64 7) -> (x .and. y?=w564:u64)
              "fine time" <- w564
              n226 = Multiply(x=u64 3600, y=w585) -> (x*y=w581:u64)
              n227 = Multiply(x=u64 60, y=w577) -> (x*y=w582:u64)
              n228 = Add(x=w582, y=w581) -> (x+y=w580:u64)
              n229 = Add(x=w580, y=w575) -> ()  [unwired: 1 out]
              n230 = Add(x=w566, y=u64 0) -> (x+y=w576:u64)
              n231 = Equal?(x=w563, y=u32 1) -> (x = y?=w594:bool)
              n232 = case shown="True" w594 {
                tunnel: w596 -> [w606 w609]
                tunnel: w576 -> [_ w608]
                tunnel: [w606 w607] -> w595
                frame False {
                }
                frame True {
                  n233 = Build Array (concatenate)(w609, w608) -> (w607:u64[])
                }
              }
              "cal 2" <- w595
              n234 = Index Array(array=w605, index=w574) -> (element=w602:u32)
              n235 = Increment(x=w602) -> (x+1=w603:u32)
              n236 = Index Array(array=w567, index (row)=w564, index (col)=w563) -> (element=w569:i64)
              n237 = Increment(x=w569) -> (x+1=w568:i64)
              n238 = Replace Array Subset(array=w605, new element=w603, index=w574) -> (w604:u32[])
              n239 = Replace Array Subset(array=w567, new element=w568, index (row)=w564, index (col)=w563) -> (w565:i64[][])
              n240 = Replace Array Subset(array=w573, new element=w566, index=w574) -> (w598:dbl[])
              n241 = case shown="True" "save data" {
                tunnel: w599 -> [_ w613]
                tunnel: w598 -> [_ w611]
                frame False {
                }
                frame True {
                  n242 = call-poly <vilib>:"Write Delimited Spreadsheet.vi"("file path (dialog if empty)"=w613, "1D data"=w611, "append to file? (new file:F)"="append csv", "delimiter (\\t)"="," ("delimiter (\\t)")) -> ()  [unwired: 10 in, 2 out]
                }
              }
              "time" <- w566
            }
          }
        }
      }
    }
    n243 = case shown="False" "RST" {
      tunnel: w251 -> [w352 _]
      tunnel: [w352 0] -> w274
      tunnel: [w351 w353] -> w272
      tunnel: w252 -> [w351 _]
      frame False {
      }
      frame True {
        n244 = Get Date/Time In Seconds() -> (seconds since 1Jan1904=w353:timestamp)
      }
    }
  }
  "error out 2" <- w62
  n245 = Close File(refnum=w54, error in=w81) -> (error out=→"error out":errorcluster)  [unwired: 1 out]
  n246 = call-poly <vilib>:"Write Delimited Spreadsheet.vi"("file path (dialog if empty)"=w65, "2D data"=w66, "append to file? (new file:F)"=FALSE, "transpose? (no:F)"=TRUE, "delimiter (\\t)"="," ("delimiter (\\t)")) -> ()  [unwired: 9 in, 2 out]
